vi "Read Power Limits (Array).vi"(8 "error in":errorcluster, 11 "Power Limits in":refnum<class "Power Limits.lvclass">) -> (0 "error out":errorcluster, 1 "Lower Power Limit":dbl[](array[numeric]), 2 "Upper Power Limit":dbl[](array[numeric]), 3 "Power Limits out":refnum<class "Power Limits.lvclass">, 4 "Changed or First Call?":bool)   [LabVIEW 2023, in "Power Limits.lvclass"]
uses:
  Power Limits.lvclass
  Power Limits.lvclass/Power Limits.ctl
  <vilib>/ADAS Replay HIL/Channels/Tag Wrapper/Polymorphic/Read Channel (Double).vi
  9f9e3b79-ae2f-4e16-acc3-d25b9e9a90ec.vi
  b0de4dd9-b279-4586-9528-e461179a1549.vi
  <vilib>/ADAS Replay HIL/Channels/Tag Wrapper/Polymorphic/Read Channel (Double).vi/b2f764de-0c1e-4784-a155-687fc995a684.vi
  <vilib>/ADAS Replay HIL/Channels/Tag Wrapper/Polymorphic/Read Channel (Double).vi/b2f764de-0c1e-4784-a155-687fc995a684.vi/c28b0ead-42ad-4072-80a2-aca7f2bd7ce3.vi
  <vilib>/ADAS Replay HIL/Channels/Tag Wrapper/Polymorphic/Read Channel (Double).vi/b2f764de-0c1e-4784-a155-687fc995a684.vi/219d0231-d98b-4193-b5cc-84f90e3c9091.vi
  <vilib>/ADAS Replay HIL/Channels/Tag Wrapper/Tag Wrapper.lvlib
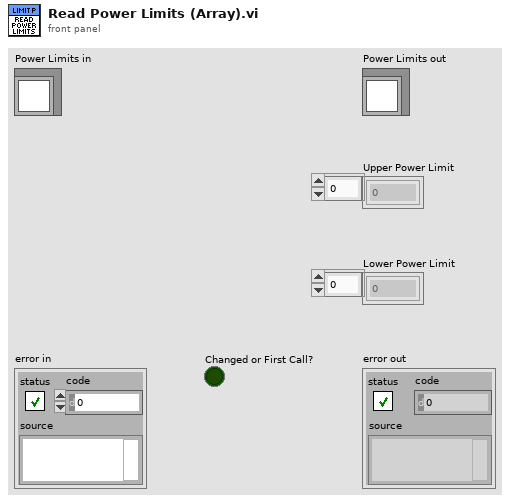
[diagram p1: front panel]
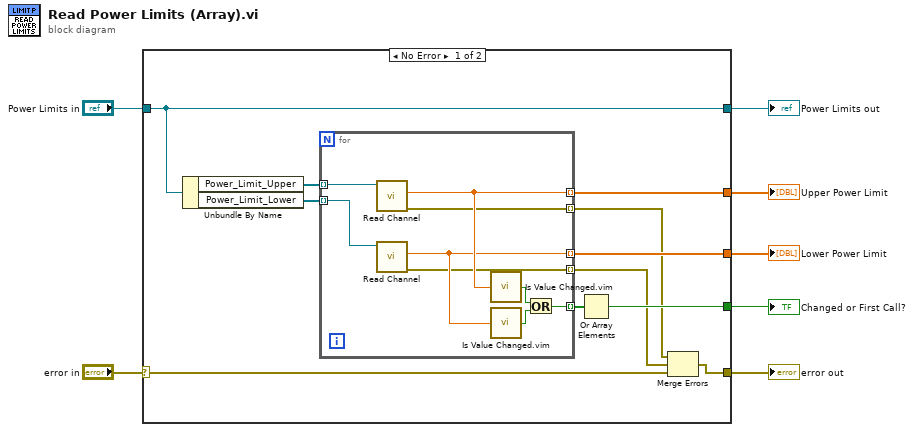
[diagram p0: block diagram]
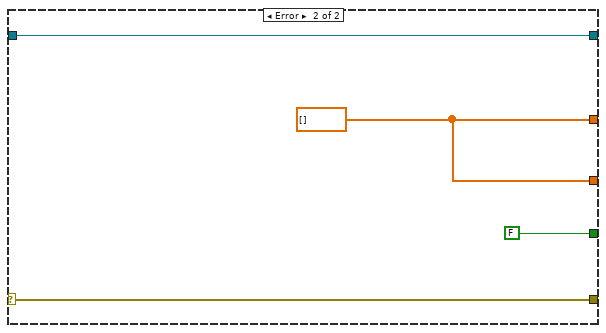
[diagram p2: hidden frame]
diagram:
  n1 = case shown="No Error" "error in" {
    selector: "error in" -> [w11 w31]
    tunnel: [w10 w31] -> w6
    tunnel: [w18 w30] -> w4
    tunnel: "Power Limits in" -> [w18 w30]
    tunnel: [w15 w28] -> w3
    tunnel: [w14 w28] -> w2
    tunnel: [w12 FALSE] -> w1
    frame No Error {
      n2 = Unbundle By Name(w18) -> ("Power_Limit_Upper"=w16:refnum<k21>[], "Power_Limit_Lower"=w17:refnum<k21>[])
      n3 = for {
        tunnel: w17 -> [w27] mode=indexing
        tunnel: w16 -> [w26] mode=indexing
        tunnel: [w22] -> w15 mode=indexing
        tunnel: [w21] -> w14 mode=indexing
        tunnel: [w23] -> w13 mode=indexing
        tunnel: [w20] -> w9 mode=indexing
        tunnel: [w19] -> w8 mode=indexing
        n4 = call-poly <vilib>:"Read Channel.vi"("ADAS HIL Channel in"=w26) -> ("error out"=w20:errorcluster, "Value out"=w22:dbl)  [unwired: 7 in, 2 out]
        n5 = call-poly <vilib>:"Read Channel.vi"("ADAS HIL Channel in"=w27) -> ("error out"=w19:errorcluster, "Value out"=w21:dbl)  [unwired: 7 in, 2 out]
        n6 = call "Is Value Changed.vim"("value"=w22) -> ("changed or first call?"=w25:bool)
        n7 = call "Is Value Changed.vim"("value"=w21) -> ("changed or first call?"=w24:bool)
        n8 = Or(x=w25, y=w24) -> (x .or. y?=w23:bool)
      }
      n9 = Or Array Elements(Boolean array=w13) -> (logical OR=w12:bool)
      n10 = Merge Errors(w9, w8, w11) -> (w10:errorcluster)
    }
    frame Error {
      w28 = dbl[] []
    }
  }
  "error out" <- w6
  "Power Limits out" <- w4
  "Upper Power Limit" <- w3
  "Lower Power Limit" <- w2
  "Changed or First Call?" <- w1
